vi "最小值计算.vi"() -> ()   [LabVIEW 2018]
uses:
  <vilib>/gmath/NI_Gmath.lvlib
panel:
  in  "formula":string caption="公式"
  in  "accuracy":dbl=1e-08 caption="精度" format="%.2e"
  in  "end":dbl=1.0 caption="结束" format="%.2f"
  in  "start":dbl caption="开始" format="%.2f"
  in  "algorithm":u16(ring) caption="算法" items=["黄金分割搜索法", "函数局部最小值（Brent法）"]
  in  "step type":u16(ring) caption="步长类型" items=["固定函数", "修正函数"]
  in  "停止":bool
  out "XY图":cluster{"Minima":dbl[], "f(Minima)":dbl[]}(graph)
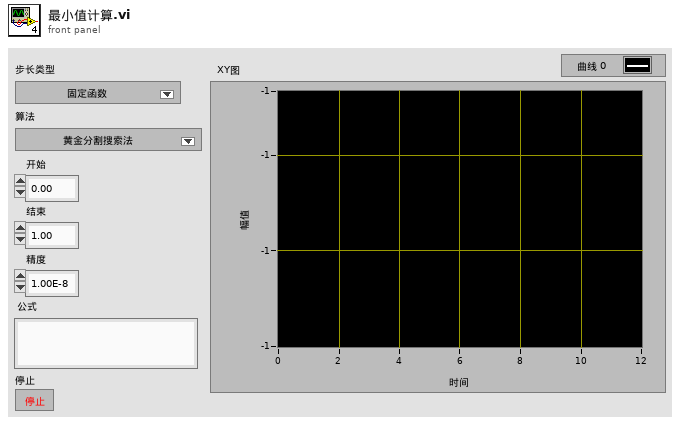
[diagram p1: front panel]
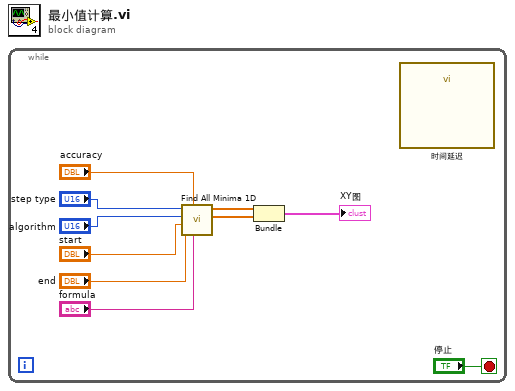
[diagram p0: block diagram]
diagram:
  n1 = while {
    stop <- "停止" stop-if-true
    n2 = call <vilib>:"Find All Minima 1D.vi"("formula"="formula", "accuracy"="accuracy", "end"="end", "start"="start", "algorithm"="algorithm", "step type"="step type") -> ("f(Minima)"=w2:dbl[], "Minima"=w3:dbl[])  [unwired: 2 out]
    n3 = Bundle("Minima"=w3, "f(Minima)"=w2) -> (→"XY图":cluster{"Minima":dbl[], "f(Minima)":dbl[]})  [unwired: 1 in]
    n4 = call "时间延迟"() -> ()  [unwired: 11 in, 1 out]
  }
